vi "Progress_Bar.vi"() -> (3 "Your Drink in Progress":u8(slide) scale=0.0..100.0)   [LabVIEW 2014]
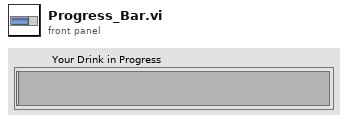
[diagram p1: front panel]
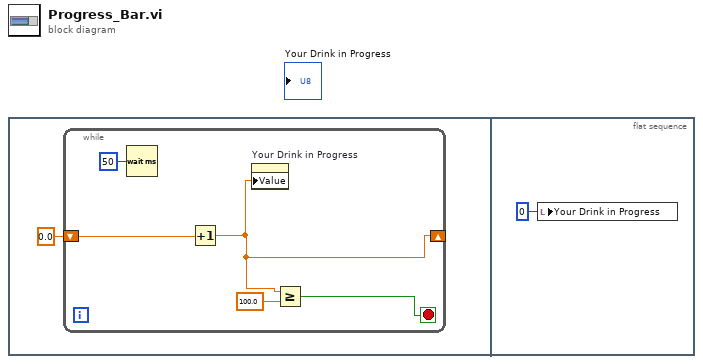
[diagram p0: block diagram]
diagram:
  n1 = flat-sequence {
    frame #0 {
      n2 = while {
        shift-right: [w2] -> _
        shift-left: 0.0 -> [w5]
        stop <- w4 stop-if-true
        n3 = Wait (ms)(milliseconds to wait=u32 50) -> ()  [unwired: 1 out]
        n4 = Increment(x=w5) -> (x+1=w2:dbl)
        n5 = property on="Your Drink in Progress" class="Slide (strict)"("Value"=w2) -> ()  [unwired: 2 in, 2 out]
        n6 = Greater Or Equal?(x=w2, y=100.0) -> (x >= y?=w4:bool)
      }
    }
    frame #1 {
      n7 = local write "Your Drink in Progress"(u8 0 ("Your Drink in Progress")) -> ()
    }
  }
